vi "Loop Frequency Counter.vi"() -> (0 "Loop Rate (Hz)":dbl format="%.2f")   [LabVIEW 2020]
doc: "Place this VI in a loop to calculate the loop rate. Using multiple copies of this VI in an application is not supported and will return incorrect results."
uses:
  <vilib>/ptbypt/NI_PtbyPt.lvlib
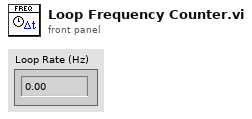
[diagram p1: front panel]
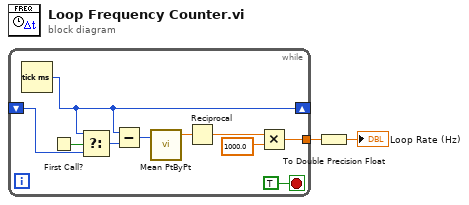
[diagram p0: block diagram]
diagram:
  n1 = while {
    shift-right: [w3] -> _
    shift-left: _ -> [w7]
    tunnel: [w4] -> w2
    stop <- TRUE stop-if-true
    n2 = Tick Count (ms)() -> (millisecond timer value=w3:u32)
    n3 = First Call?() -> (First Call?: T/F=w12:bool)
    n4 = Select(t=w3, s=w12, f=w7) -> (s? t:f=w11:u32)
    n5 = Subtract(x=w3, y=w11) -> (x-y=w10:u32)
    n6 = call <vilib>:"Mean PtByPt.vi"("x"=w10) -> ("mean"=w9:dbl)  [unwired: 3 in, 1 out]
    n7 = Reciprocal(x=w9) -> (1/x=w5:dbl)
    n8 = Multiply(x=w5, y=1000.0) -> (x*y=w4:dbl)
  }
  n9 = To Double Precision Float(number=w2) -> (double precision float=→"Loop Rate (Hz)":dbl)
